vi "Launch Remote Control.vi"(8 "error in":errorcluster, 11 "Master Controller in":refnum<class "EMS User Interface.lvclass">) -> (0 "error out":errorcluster, 3 "Master Controller out":refnum<class "EMS User Interface.lvclass">)   [LabVIEW 2018, in "EMS User Interface Actor.lvlib" / "EMS User Interface.lvclass"]
uses:
  EMS User Interface.lvclass
  C:/Users/Administrator/Desktop/2018LabVIEW EMS/EMS Generic Actor/EMS Generic/EMS Generic.lvclass
  C:/Program Files (x86)/National Instruments/LabVIEW 2018/vi.lib/ActorFramework/Actor/Actor.lvclass
  Remote Operation/Alabama Power Remote Actor/Alabama Power Remote/Alabama Power Remote.lvclass
  C:/Users/Administrator/Desktop/2018LabVIEW EMS/Remote Operation/Remote Operation Abstract/Remote Operation Abstract.lvclass
  EMS User Interface Messages/Remote Activate Msg/Remote Activate Msg.lvclass
  C:/Users/Administrator/Desktop/2018LabVIEW EMS/Remote Operation/Remote Operation Abstract Messages/Activate Microgrid Msg/Activate Microgrid Msg.lvclass
  EMS User Interface Messages/Remote Blackstart Msg/Remote Blackstart Msg.lvclass
  C:/Users/Administrator/Desktop/2018LabVIEW EMS/Remote Operation/Remote Operation Abstract Messages/Blackstart Microgrid Msg/Blackstart Microgrid Msg.lvclass
  EMS User Interface Messages/Remote Island Msg/Remote Island Msg.lvclass
  C:/Users/Administrator/Desktop/2018LabVIEW EMS/Remote Operation/Remote Operation Abstract Messages/Island Microgrid Msg/Island Microgrid Msg.lvclass
  EMS User Interface Messages/Remote Resynch Msg/Remote Resynch Msg.lvclass
  C:/Users/Administrator/Desktop/2018LabVIEW EMS/Remote Operation/Remote Operation Abstract Messages/Resynchronize Microgrid Msg/Resynchronize Microgrid Msg.lvclass
  EMS User Interface Messages/Remote Shutdown Msg/Remote Shutdown Msg.lvclass
  C:/Users/Administrator/Desktop/2018LabVIEW EMS/Remote Operation/Remote Operation Abstract Messages/Shutdown Microgrid Msg/Shutdown Microgrid Msg.lvclass
  EMS User Interface Messages/Remote Start Msg/Remote Start Msg.lvclass
  C:/Users/Administrator/Desktop/2018LabVIEW EMS/Remote Operation/Remote Operation Abstract Messages/Start Microgrid Msg/Start Microgrid Msg.lvclass
  EMS User Interface Messages/Remote Stop Msg/Remote Stop Msg.lvclass
  C:/Users/Administrator/Desktop/2018LabVIEW EMS/Remote Operation/Remote Operation Abstract Messages/Stop Microgrid Msg/Stop Microgrid Msg.lvclass
  Remote Operation/Remote Operation Abstract/Remote Operation Abstract.lvclass/Remote Operation Abstract.ctl
  EMS User Interface.lvclass/EMS User Interface.ctl
  Remote Operation/Remote Operation Abstract/Remote Operation Abstract.lvclass
  <vilib>/ActorFramework/Actor/Actor.lvclass
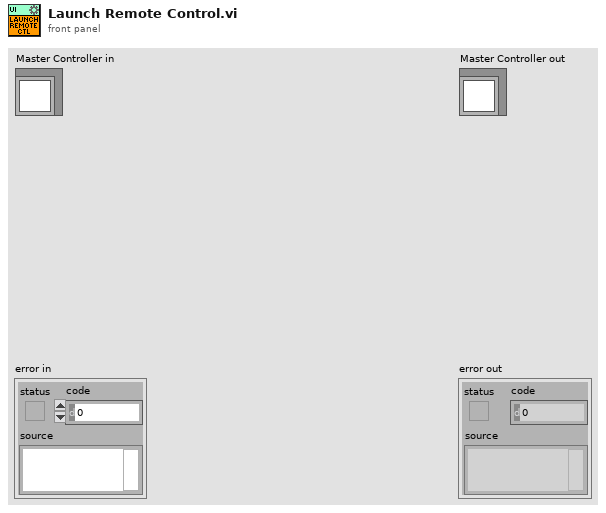
[diagram p1: front panel]
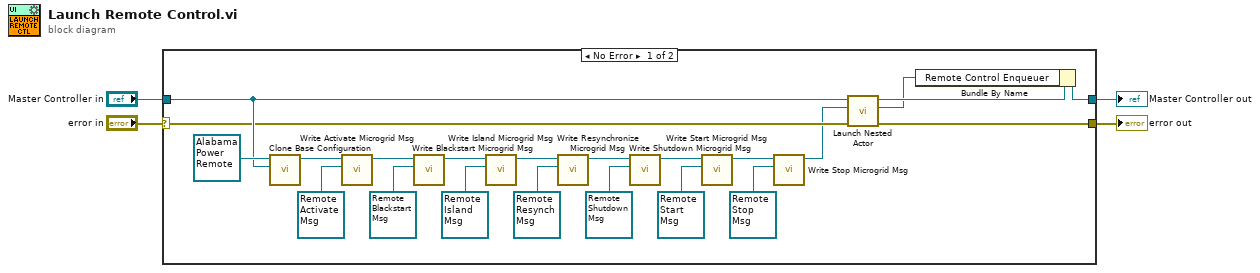
[diagram p0: block diagram]
diagram:
  n1 = case shown="No Error" "error in" {
    selector: "error in" -> [w9 w28]
    tunnel: [w8 w28] -> w3
    tunnel: [w6 w27] -> w1
    tunnel: "Master Controller in" -> [w11 w27]
    frame No Error {
      n2 = call-dynamic "Clone Base Configuration.vi"("Source Object"=w11, "Target Object in"=refnum<class "Alabama Power Remote.lvclass"> refnum ("Alabama Power Remote Actor.lvlib:Alabama Power Remote.lvclass")) -> ("Target Object out"=w25:refnum<class "Alabama Power Remote.lvclass">)  [unwired: 9 in]
      n3 = call "Write Activate Microgrid Msg.vi"("Activate Microgrid Msg"=refnum<class "Remote Activate Msg.lvclass"> refnum ("Master Controller Core.lvlib:Remote Activate Msg.lvclass"), "Remote Operation Abstract in"=w25) -> ("Remote Operation Abstract out"=w24:refnum<class "Alabama Power Remote.lvclass">)  [unwired: 9 in]
      n4 = call "Write Blackstart Microgrid Msg.vi"("Blackstart Microgrid Msg"=refnum<class "Remote Blackstart Msg.lvclass"> refnum ("Master Controller Core.lvlib:Remote Blackstart Msg.lvclass"), "Remote Operation Abstract in"=w24) -> ("Remote Operation Abstract out"=w23:refnum<class "Alabama Power Remote.lvclass">)  [unwired: 9 in]
      n5 = call "Write Island Microgrid Msg.vi"("Island Microgrid Msg"=refnum<class "Remote Island Msg.lvclass"> refnum ("Master Controller Core.lvlib:Remote Island Msg.lvclass"), "Remote Operation Abstract in"=w23) -> ("Remote Operation Abstract out"=w22:refnum<class "Alabama Power Remote.lvclass">)  [unwired: 9 in]
      n6 = call "Write Resynchronize Microgrid Msg.vi"("Resynchronize Microgrid Msg"=refnum<class "Remote Resynch Msg.lvclass"> refnum ("Master Controller Core.lvlib:Remote Resynch Msg.lvclass"), "Remote Operation Abstract in"=w22) -> ("Remote Operation Abstract out"=w21:refnum<class "Alabama Power Remote.lvclass">)  [unwired: 9 in]
      n7 = call "Write Shutdown Microgrid Msg.vi"("Shutdown Microgrid Msg"=refnum<class "Remote Shutdown Msg.lvclass"> refnum ("Master Controller Core.lvlib:Remote Shutdown Msg.lvclass"), "Remote Operation Abstract in"=w21) -> ("Remote Operation Abstract out"=w20:refnum<class "Alabama Power Remote.lvclass">)  [unwired: 9 in]
      n8 = call "Write Start Microgrid Msg.vi"("Start Microgrid Msg"=refnum<class "Remote Start Msg.lvclass"> refnum ("Master Controller Core.lvlib:Remote Start Msg.lvclass"), "Remote Operation Abstract in"=w20) -> ("Remote Operation Abstract out"=w19:refnum<class "Alabama Power Remote.lvclass">)  [unwired: 9 in]
      n9 = call "Write Stop Microgrid Msg.vi"("Stop Microgrid Msg"=refnum<class "Remote Stop Msg.lvclass"> refnum ("Master Controller Core.lvlib:Remote Stop Msg.lvclass"), "Remote Operation Abstract in"=w19) -> ("Remote Operation Abstract out"=w7:refnum<class "Alabama Power Remote.lvclass">)  [unwired: 9 in]
      n10 = call <vilib>:"Launch Nested Actor.vi"("error in (no error)"=w9, "Nested Actor"=w7, "Caller Actor in"=w11) -> ("error out"=w8:errorcluster, "Nested Actor's Enqueuer"=w5:refnum<class "Message Enqueuer.lvclass">, "Caller Actor out"=w10:refnum<class "EMS User Interface.lvclass">)  [unwired: 6 in]
      n11 = Bundle By Name(cluster=w10, "Remote Control Enqueuer"=w5) -> (w6:refnum<class "EMS User Interface.lvclass">)
    }
    frame Error {
    }
  }
  "error out" <- w3
  "Master Controller out" <- w1
